vi "triggerAcquisition.vi"() -> (0 "return type":i32)   [LabVIEW 2012]
uses:
  hidapi_32bits.dll
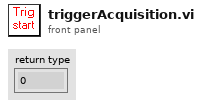
[diagram p1: front panel]
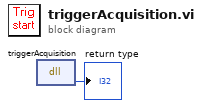
[diagram p0: block diagram]
diagram:
  n1 = dll-call lib="C:/All_Data/mikrocont/Project1/New_controller__Jan_2015/LabView_Aug_2015/hidapi_32bits.dll" fn="triggerAcquisition"() -> ("return type"=→"return type":i32)  [unwired: 3 in, 2 out]
